vi "Update Fire.vi"(8 "error in (no error)":errorcluster, 10 "Fire (%)":dbl, 11 "Kitchen Actor in":refnum<class "Kitchen Actor.lvclass">) -> (0 "error out":errorcluster, 3 "Kitchen Actor out":refnum<class "Kitchen Actor.lvclass">)   [LabVIEW 2024, in "Kitchen Actor.lvlib" / "Kitchen Actor.lvclass"]
uses:
  Kitchen Actor.lvclass
  Kitchen Actor.lvclass/Kitchen Actor.ctl
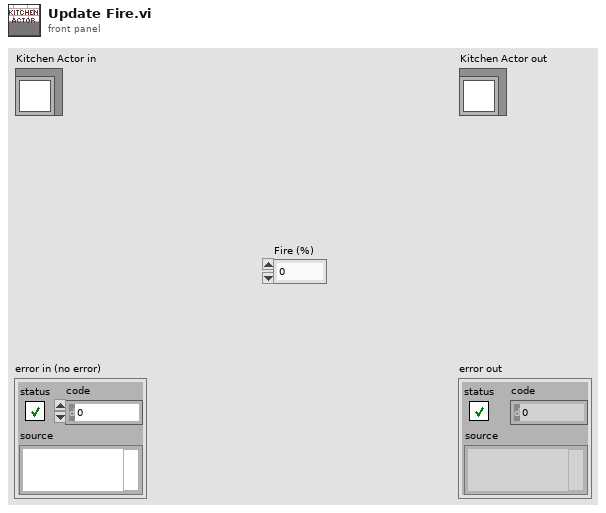
[diagram p1: front panel]
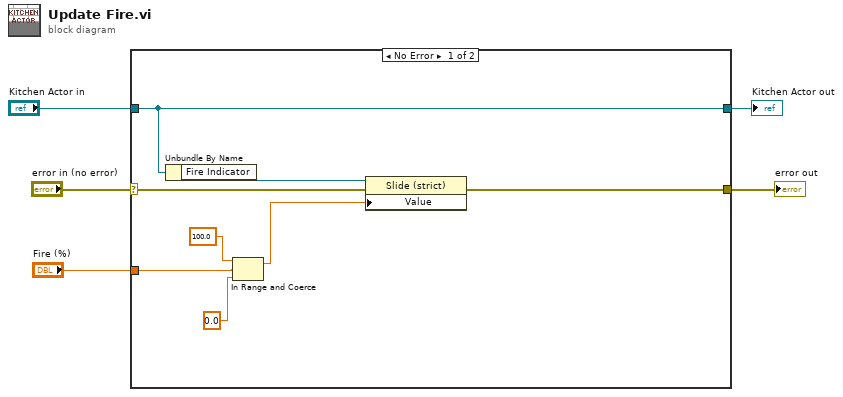
[diagram p0: block diagram]
diagram:
  n1 = case shown="No Error" "error in (no error)" {
    selector: "error in (no error)" -> [w13 w15]
    tunnel: [w11 w15] -> w4
    tunnel: [w12 w14] -> w2
    tunnel: "Kitchen Actor in" -> [w12 w14]
    tunnel: "Fire (%)" -> [w6 _]
    frame No Error {
      n2 = Unbundle By Name(w12) -> ("Fire Indicator"=w10:refnum<vi>)
      n3 = In Range and Coerce(upper limit=100.0, x=w6, lower limit=0.0) -> (coerced(x)=w9:dbl)  [unwired: 1 out]
      n4 = property class="Slide (strict)"(reference=w10, error in=w13, "Value"=w9) -> (error out=w11:errorcluster)  [unwired: 1 out]
    }
    frame Error {
    }
  }
  "error out" <- w4
  "Kitchen Actor out" <- w2
